vi "List Available Phidgets.vi"(10 "Timeout":u32=500) -> (0 "error out":errorcluster, 3 "Available Handles":u64[](array[numeric]))   [LabVIEW 2012, in "Phidget Manager.lvlib"]
doc: "Lists Phidgets that are available to your system. Be sure to clean up after this call using Release All.vi\n\nSpecifically, List Phidgets.vi will give you a list of Phidget IDs that you can use to\nget information about the attached Phidgets.\n\nDo not use these IDs to open Phidgets directly, though you can use \nCommon requests such as getDeviceInfo to get all the information\nneeded to open that Phidget separately.\n\nOnce you are done, remember to clean up the list of temperary\nreferences using Release All.vi"
uses:
  <instrlib>/Phidgets/Phidget Manager/Phidget Manager.lvlib
  <instrlib>/Phidgets/Phidget Common/Phidget Common.lvlib
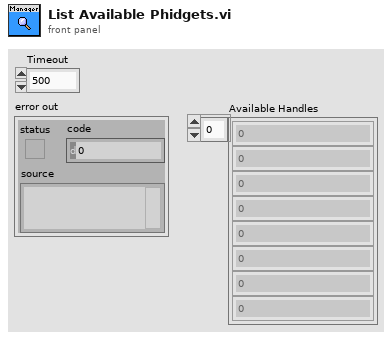
[diagram p1: front panel]
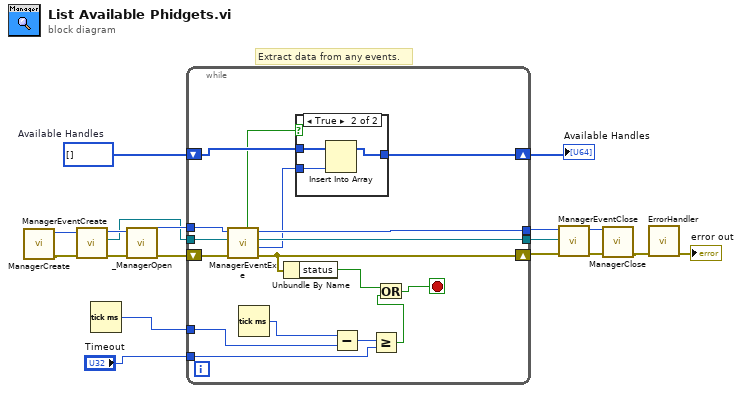
[diagram p0: block diagram]
diagram:
  w14 = u64[] []  # Available Handles
  # "Extract data from any events."
  n1 = call <instrlib>:"ManagerCreate.vi"() -> ("error out"=w12:errorcluster, "Device Out"=w6:u64)  [unwired: 10 in]
  n2 = call <instrlib>:"ManagerEventCreate.vi"("error in (no error)"=w12, "Manager In"=w6) -> ("error out"=w10:errorcluster, "Event Registration Refnum"=w7:refnum<event-registration>, "Manager Out"=w11:u64)  [unwired: 7 in]
  n3 = Tick Count (ms)() -> (millisecond timer value=w15:u32)
  n4 = call <instrlib>:"_ManagerOpen.vi"("error in"=w10, "Device In"=w11) -> ("error out"=w9:errorcluster, "Device Out"=w8:u64)  [unwired: 8 in]
  n5 = while {
    tunnel: w8 -> [w35]
    tunnel: w7 -> [w31]
    tunnel: [w34] -> w2
    shift-right: [w22] -> w17
    shift-left: w9 -> [w33]
    tunnel: [w32] -> w16
    tunnel: w15 -> [w30]
    shift-right: [w24] -> w13
    shift-left: w14 -> [w25]
    tunnel: "Timeout" -> [w20]
    stop <- w26 stop-if-true
    n6 = call <instrlib>:"ManagerEventExe.vi"("error in (no error)"=w33, "Event Registration Refnum In"=w31, "Manager In"=w35) -> ("error out"=w22:errorcluster, "phid"=w23:u64, "Event Registration Refnum Out"=w34:refnum<event-registration>, "Manager Out"=w32:u64, "Event?"=w21:bool)  [unwired: 3 in, 1 out]
    n7 = Tick Count (ms)() -> (millisecond timer value=w29:u32)
    n8 = Unbundle By Name(w22) -> ("status"=w19:bool)
    n9 = case shown="True" w21 {
      tunnel: w25 -> [w36 w39]
      tunnel: [w36 w38] -> w24
      tunnel: w23 -> [_ w37]
      frame False {
      }
      frame True {
        n10 = Insert Into Array(array=w39, new element=w37) -> (w38:u64[])  [unwired: 1 in]
      }
    }
    n11 = Subtract(x=w29, y=w30) -> (x-y=w28:u32)
    n12 = Greater Or Equal?(x=w28, y=w20) -> (x >= y?=w27:bool)
    n13 = Or(x=w19, y=w27) -> (x .or. y?=w26:bool)
  }
  "Available Handles" <- w13
  n14 = call <instrlib>:"ManagerEventClose.vi"("error in (no error)"=w17, "Event Registration Refnum In"=w2, "Manager In"=w16) -> ("error out"=w4:errorcluster, "Manager Out"=w5:u64)  [unwired: 7 in]
  n15 = call <instrlib>:"ManagerClose.vi"("error in"=w4, "Manager In"=w5) -> ("error out"=w3:errorcluster)  [unwired: 9 in]
  n16 = call <instrlib>:"ErrorHandler.vi"("error in"=w3) -> ("error out"=→"error out":errorcluster)  [unwired: 9 in, 1 out]
